vi "Vibrator_Test.vi"() -> ()   [LabVIEW 2016]
uses:
  <vilib>/Platform/TimedLoop/XDataNode/timing_clust.ctl
  <vilib>/Platform/TimedLoop/XDataNode/nitl_modes.ctl
  <vilib>/Platform/TimedLoop/XDataNode/wakeup.ctl
  <vilib>/Utility/error.llb/Error Cluster From Error Code.vi
  <vilib>/myRIO/Common/Instrument Driver Framework/myRIO v1.0/PWM/vis/myRIO v1.0 Write PWM.vi
  <vilib>/Platform/TimedLoop/XDataNode/XDataNode.xnode
  <vilib>/Platform/TimedLoop/XDataNode/XDNodeRunTimeDep.lvlib
  <vilib>/myRIO/Instrument Drivers/Onboard IO/PWM/PWM.lvlib
panel:
  out "Finished Late?":bool
  out "error out":errorcluster
  in  "Duty Cycle":dbl(slide) scale=0.0..1.0
  in  "stop":bool
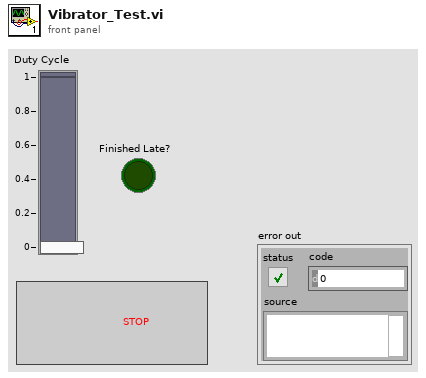
[diagram p1: front panel]
types:
  T1 = typedef "PWM.lvlib/PWM Reference.ctl" = cluster{"myRIO Reference":T2, "PWM Channels Enum":T6, "PWM Configuration":T7}
  T2 = typedef "myRIO Generic Hardware Reference.ctl" = cluster{"myRIO Model":T3, "myRIO Hardware Reference":T4}
  T3 = typedef "Hardware Version Enum.ctl" = enum16{"Unknown", "myRIO-1900", "myRIO-1950", "roboRIO", "NI ELVIS RIO CM"}
  T4 = typedef "myRIO v1.0 Reference.ctl" = cluster{"Generic FPGA Reference":T5, "Allow multiple opens":bool}
  T5 = typedef "Generic FPGA Reference.ctl" = refnum<k20>
  T6 = typedef "PWM Channels Enum.ctl" = enum16{"Not Connected", "C/PWM0", "C/PWM1", "A/PWM0", "A/PWM1", "A/PWM2", "B/PWM0", "B/PWM1", "B/PWM2", "PWM/PWM0", "PWM/PWM1", "PWM/PWM2", "PWM/PWM3", "PWM/PWM4", "PWM/PWM5", "PWM/PWM6", "PWM/PWM7", "PWM/PWM8", "PWM/PWM9"}
  T7 = typedef "PWM.lvlib/PWM Configuration.ctl" = cluster{"Frequency":dbl, "Duty Cycle":dbl}
  T8 = typedef "XDNodeRunTimeDep.lvlib/timing_clust.ctl" = cluster{"Expected End [f-1]":u64, "Actual End [f-1]":u64, "Finished Late? [f-1]":bool, "Expected End [i-1]":u64, "Actual End [i-1]":u64, "Finished Late? [i-1]":bool, "Expected Start [i]":u64, "Actual Start [i]":u64, "Expected Start [f]":u64, "Actual Start [f]":u64, "Source Name":string, "Structure Name":string, "Period":i64, "Deadline":i64, "Offset":i64, "Start":i64, "Priority":i32, "Timeout":i32, "Mode":T9, "Wakeup Reason":T10, "Error":errorcluster, "Source Type":string, "Secondary Source Type":string, "Global End Time":u64, "Global Start Time":u64, "Frame Duration":u64, "Iteration Duration":u64, "Assigned CPU":i32, "I/O Scan Engine Mode":u32}
  T9 = typedef "XDNodeRunTimeDep.lvlib/nitl_modes.ctl" = enum32{"No Change", "Process missed periods, maintain original phase", "Discard missed periods, maintain original phase", "Process missed periods, ignore original phase", "Discard missed periods, ignore original phase"}
  T10 = typedef "XDNodeRunTimeDep.lvlib/wakeup.ctl" = enum32{"Normal", "Aborted", "Asynchronous wakeup", "Timing source error", "Timed loop error", "Timeout"}
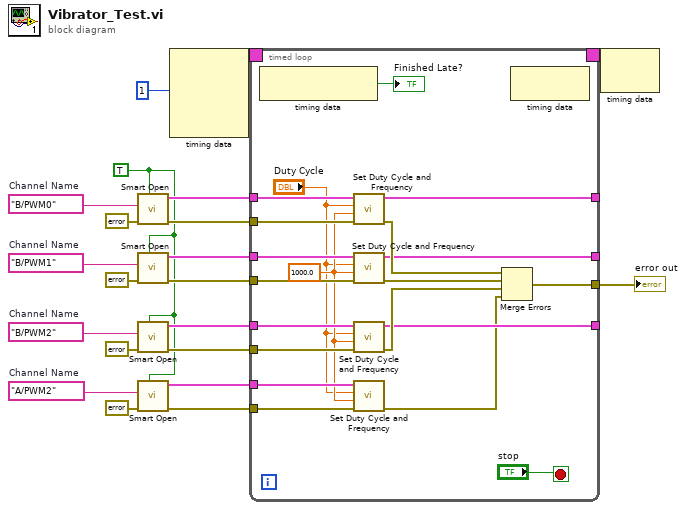
[diagram p0: block diagram]
diagram:
  w2 = tag "A/PWM2"  # Channel Name
  w1 = TRUE ("Allow multiple opens?")
  w10 = tag "B/PWM2"  # Channel Name
  w13 = tag "B/PWM1"  # Channel Name
  w18 = tag "B/PWM0"  # Channel Name
  n1 = call <vilib>:"Smart Open.vi"("Allow multiple opens?"=w1, "error in (no error)"=errorcluster {"status"=FALSE, "code"=0, "source"=""}, "Channel Name"=w18) -> ("error out"=w16:errorcluster, "PWM Ref Out"=w17:T1)  [unwired: 7 in]
  n2 = call <vilib>:"Smart Open.vi"("Allow multiple opens?"=w1, "error in (no error)"=errorcluster {"status"=FALSE, "code"=0, "source"=""}, "Channel Name"=w13) -> ("error out"=w11:errorcluster, "PWM Ref Out"=w12:T1)  [unwired: 7 in]
  n3 = call <vilib>:"Smart Open.vi"("Allow multiple opens?"=w1, "error in (no error)"=errorcluster {"status"=FALSE, "code"=0, "source"=""}, "Channel Name"=w10) -> ("error out"=w7:errorcluster, "PWM Ref Out"=w8:T1)  [unwired: 7 in]
  n4 = call <vilib>:"Smart Open.vi"("Allow multiple opens?"=w1, "error in (no error)"=errorcluster {"status"=FALSE, "code"=0, "source"=""}, "Channel Name"=w2) -> ("error out"=w5:errorcluster, "PWM Ref Out"=w4:T1)  [unwired: 7 in]
  n5 = node-c288(i64 1 ("Period")) -> (w21:T8)  [unwired: 3 in]
  n6 = timed-loop {
    timing: w21 -> [_]
    timing-out: [_] -> w20
    tunnel: w17 -> [w40]
    tunnel: w16 -> [w39]
    tunnel: w12 -> [w38]
    tunnel: w11 -> [w37]
    tunnel: w8 -> [w36]
    tunnel: w7 -> [w35]
    tunnel: [w31] -> w6
    tunnel: [w30] -> _
    tunnel: [w29] -> _
    tunnel: [w28] -> _
    tunnel: w4 -> [w25]
    tunnel: w5 -> [w26]
    stop <- "stop" stop-if-true
    w24 = 1000.0 ("Frequency [Hz]")
    n7 = node-c288() -> (→"Finished Late?":bool)  [unwired: 1 in]
    n8 = call <vilib>:"Set Duty Cycle and Frequency.vi"("error in (no error)"=w39, "Frequency [Hz]"=w24, "Duty Cycle"="Duty Cycle", "PWM Ref In"=w40) -> ("error out"=w34:errorcluster, "PWM Ref Out"=w30:T1)  [unwired: 5 in]
    n9 = call <vilib>:"Set Duty Cycle and Frequency.vi"("error in (no error)"=w37, "Frequency [Hz]"=w24, "Duty Cycle"="Duty Cycle", "PWM Ref In"=w38) -> ("error out"=w33:errorcluster, "PWM Ref Out"=w29:T1)  [unwired: 5 in]
    n10 = call <vilib>:"Set Duty Cycle and Frequency.vi"("error in (no error)"=w35, "Frequency [Hz]"=w24, "Duty Cycle"="Duty Cycle", "PWM Ref In"=w36) -> ("error out"=w32:errorcluster, "PWM Ref Out"=w28:T1)  [unwired: 5 in]
    n11 = call <vilib>:"Set Duty Cycle and Frequency.vi"("error in (no error)"=w26, "Frequency [Hz]"=w24, "Duty Cycle"="Duty Cycle", "PWM Ref In"=w25) -> ("error out"=w22:errorcluster)  [unwired: 5 in, 1 out]
    n12 = Merge Errors(w34, w33, w32, w22) -> (w31:errorcluster)
    n13 = node-c288() -> ()  [unwired: 1 in, 1 out]
  }
  "error out" <- w6
  n14 = node-c288(w20) -> ()  [unwired: 1 out]
